vi "Perform Action.vi"(8 "error in":errorcluster, 10 "Input":variant, 11 "Control Load CFG in":refnum<class "EL Control Load CFG.lvclass">) -> (0 "error out":errorcluster, 2 "Output":variant, 3 "Control Load CFG out":refnum<class "EL Control Load CFG.lvclass">)   [LabVIEW 2024, in "EL Control Load CFG.lvclass"]
uses:
  EL Control Load CFG.lvclass
  SCPI PE Input.ctl
  EL Control Load CFG.lvclass/EL Control Load CFG.ctl
  <userlib>/_OpenG.lib/time/time.llb/openg_time.lvlib
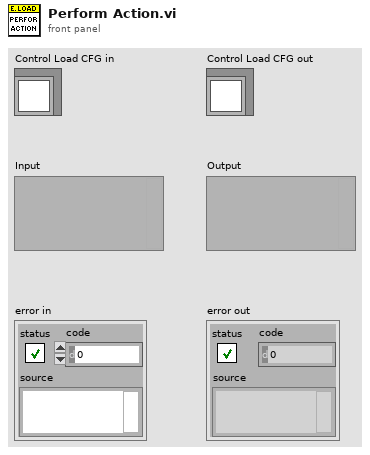
[diagram p1: front panel]
types:
  T1 = typedef "SCPI PE Input.ctl" = cluster{"Action":enum16{"Write", "Query"}, "SCPI":string}
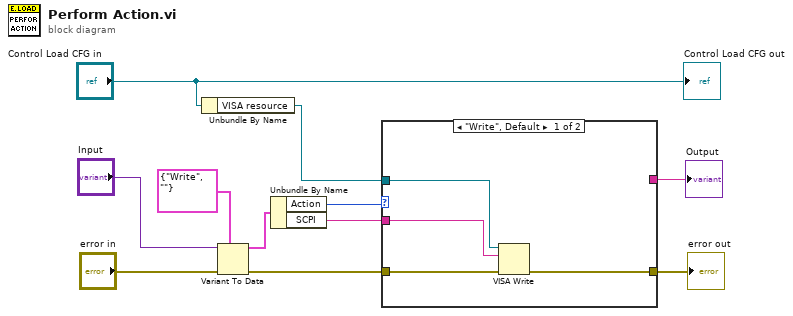
[diagram p0: block diagram]
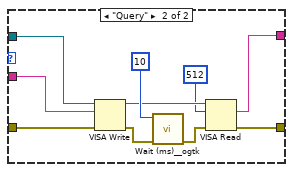
[diagram p2: hidden frame]
diagram:
  n1 = Unbundle By Name("Control Load CFG in") -> ("VISA resource"=w6:refnum<visa-resource-name>)
  n2 = Variant To Data(error in="error in", type=T1 {"Action"=enum."Write", "SCPI"=""} ("PE Input"), Variant="Input") -> (data=w8:T1, error out=w4:errorcluster)
  n3 = Unbundle By Name(w8) -> ("Action"=w7:enum16{"Write", "Query"}, "SCPI"=w5:string)
  n4 = case shown="\"Write\", Default" w7 {
    tunnel: w6 -> [w13 w23]
    tunnel: w5 -> [w12 w24]
    tunnel: w4 -> [w15 w25]
    tunnel: [w14 w19] -> w3
    tunnel: [_ w16] -> w1
    frame "Write", Default {
      n5 = VISA Write(VISA resource name=w13, write buffer=w12, error in (no error)=w15) -> (error out=w14:errorcluster)  [unwired: 2 out]
    }
    frame "Query" {
      n6 = VISA Write(VISA resource name=w23, write buffer=w24, error in (no error)=w25) -> (VISA resource name out=w18:refnum<visa-resource-name>, error out=w22:errorcluster)  [unwired: 1 out]
      n7 = call <userlib>:"Wait (ms)__ogtk.vi"("error in (no error)"=w22, "milliseconds to wait"=u32 10) -> ("error out"=w20:errorcluster)  [unwired: 8 in, 1 out]
      n8 = VISA Read(VISA resource name=w18, byte count=u32 512, error in (no error)=w20) -> (read buffer=w16:string, error out=w19:errorcluster)  [unwired: 2 out]
    }
  }
  "error out" <- w3
  "Output" <- w1
  "Control Load CFG out" <- "Control Load CFG in"
